vi "XLP80_CAN_CVM.vi"(7 "Function":string, 8 "err in":errorcluster caption="error") -> (0 "err out":errorcluster caption="error")   [LabVIEW 2021]
uses:
  XLP80_FGlob/1886_FGlob_TDefs_Enum_FGlobItems.ctl
  XLP80_Globals/Globals_Settings_XLP80.vi
  XLP80_Globals/XLP80_Globals_Status.vi
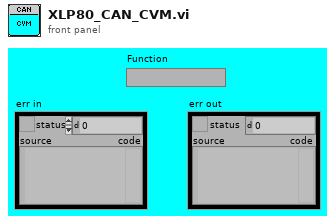
[diagram p1: front panel]
types:
  T1 = cluster{"CVM Graph":cluster{"CVM Warning":sgl, "CVM Alarm":sgl, "CVM GraphMin":sgl, "CVM GraphMax":sgl}, "Cells":i32, "StartChannel":string, "CVM Simulate":bool, "CVMSimulation":cluster{"CVMin":sgl, "CVPeakNoise":sgl}}
  T2 = typedef "1886_FGlob_TDefs_Enum_FGlobItems.ctl" = enum16{"Put one", "Put all", "Recall one", "Recall all"}
  T3 = typedef "XLP80_Action_TDefEnumControl.ctl" = enum16{"Testmode_A", "Testmode_B"}
  T4 = cluster{"Signal Name":string[], "Description":string[], "Unit":string[], "Min":dbl[], "Max":dbl[], "HV & Software":bool[], "Basis Funktion":bool[], "Power Management":bool[], "OperationMode":bool[], "Shutdown":bool[], "Alarm":bool[], "LogEnable":bool[]}
  T5 = cluster{"Signal Name":string[], "Description":string[], "Unit":string[], "Min":dbl[], "Max":dbl[], "TestmodeA":bool[], "LogEnable":bool[]}
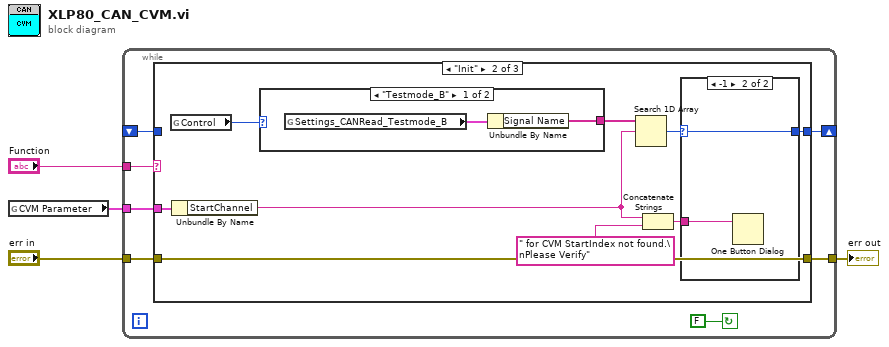
[diagram p0: block diagram]
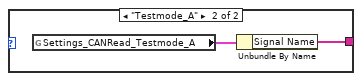
[diagram p4: hidden frame]
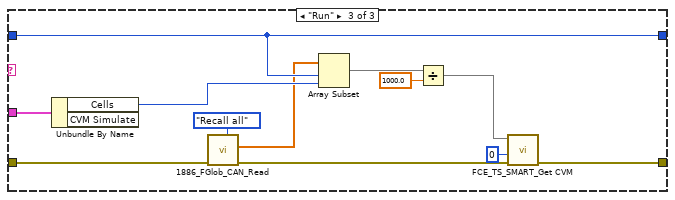
[diagram p5: hidden frame]
diagram:
  n1 = global read "Globals_Settings_XLP80.vi" "CVM Parameter"() -> (w2:T1)
  n2 = while {
    tunnel: "Function" -> [w10]
    tunnel: "err in" -> [w9]
    tunnel: w2 -> [w8]
    shift-right: [w7] -> _
    shift-left: _ -> [w6]
    tunnel: [w5] -> w1
    stop <- FALSE continue-if-true
    n3 = case shown="\"Init\"" w10 {
      tunnel: w9 -> [w12 w14 w40]
      tunnel: w8 -> [_ w22 w41]
      tunnel: [w13 w15 w38] -> w7
      tunnel: w6 -> [w13 _ w38]
      tunnel: [w12 w14 w34] -> w5
      frame Default {
      }
      frame "Init" {
        n4 = global read "XLP80_Globals_Status.vi" "Control"() -> (w21:T3)
        n5 = Unbundle By Name(w22) -> ("StartChannel"=w18:string)
        n6 = case shown="\"Testmode_B\"" w21 {
          tunnel: [w26 w28] -> w20
          frame "Testmode_B" {
            n7 = global read "Globals_Settings_XLP80.vi" "Settings_CANRead_Testmode_B"() -> (w27:T4)
            n8 = Unbundle By Name(w27) -> ("Signal Name"=w26:string[])
          }
          frame "Testmode_A" {
            n9 = global read "Globals_Settings_XLP80.vi" "Settings_CANRead_Testmode_A"() -> (w29:T5)
            n10 = Unbundle By Name(w29) -> ("Signal Name"=w28:string[])
          }
        }
        n11 = Search 1D Array(1D array=w20, element=w18) -> (index of element=w19:i32)  [unwired: 1 in]
        n12 = Concatenate Strings(w18, " for CVM StartIndex not found.\nPlease Verify" ("string")) -> (w16:string)
        n13 = case shown="-1" w19 {
          selector: w19 -> [w23 w24]
          tunnel: w16 -> [_ w25]
          tunnel: [w23 w24] -> w15
          frame 0, Default {
          }
          frame -1 {
            n14 = One Button Dialog(message=w25) -> ()  [unwired: 1 in, 1 out]
          }
        }
      }
      frame "Run" {
        n15 = Unbundle By Name(w41) -> ("Cells"=w39:i32)  [unwired: 1 out]
        n16 = call "1886_FGlob_CAN_Read.vi"("Function (Recall One)"=1886_FGlob_TDefs_Enum_FGlobItems."Recall all", "err in"=w40) -> ("err out"=w35:errorcluster, "AI Values OUT"=w36:dbl[])  [unwired: 7 in, 1 out]
        n17 = Array Subset(array=w36, index=w38, length=w39) -> (w32:dbl[])
        n18 = Divide(x=w32, y=1000.0 ("values")) -> (x/y=w31:dbl[])
        n19 = call "FCE_TS_SMART_Get CVM.vi"("err in"=w35, "Delay (0)"=0, "CVM Data IN"=w31) -> ("err out"=w34:errorcluster)  [unwired: 8 in]
      }
    }
  }
  "err out" <- w1
